vi "LABVIEW做的蓝牙数据发送程序.vi"() -> ()   [LabVIEW 2018]
panel:
  in  "蓝牙设备列表":i32(listbox)
  in  "停止":bool
  out "数据输出":string="SND: AT SP 6\nRCV: AT SP 6\nOK\r\r>SND: AT DP\nRCV: AT DP\nISO 15765-4 (CAN 11/500)\r\r>SND: 01 00\nRCV: 01 00\n41 00 BE 1F B8 10 \r\r>SND: AT H1\nRCV: AT H1\nOK\r\r>SND: 01 00\nRCV: 01 00\n7E1 06 41 00 BE 1F B8 10 \r\r>"
  in  "服务列表":i32(listbox)
  in  "send":bool
  in  "数据输入":string
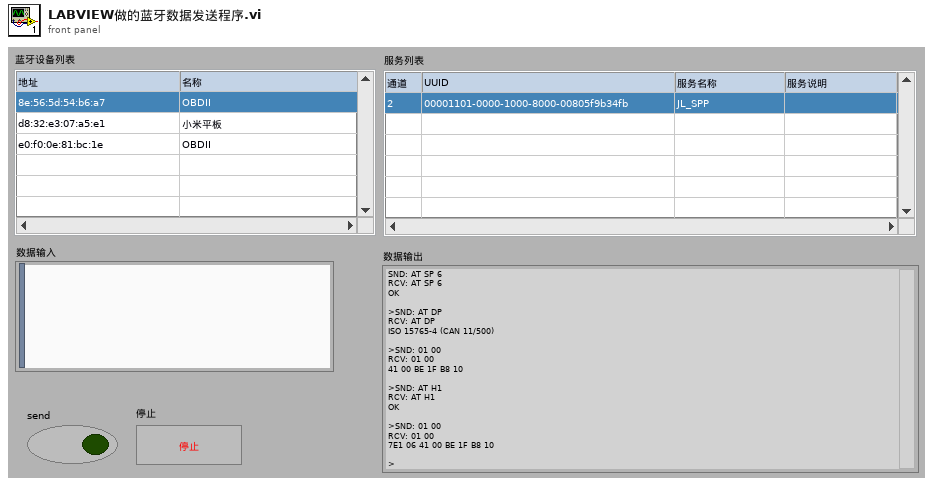
[diagram p1: front panel]
types:
  T1 = cluster{"Address":string, "Device Name":string}[]
  T2 = cluster{"channel":u16, "uuid":string, "service name":string, "service description":string}[]
  T3 = cluster{"channel":u16, "uuid":string, "service name":string, "service description":string}
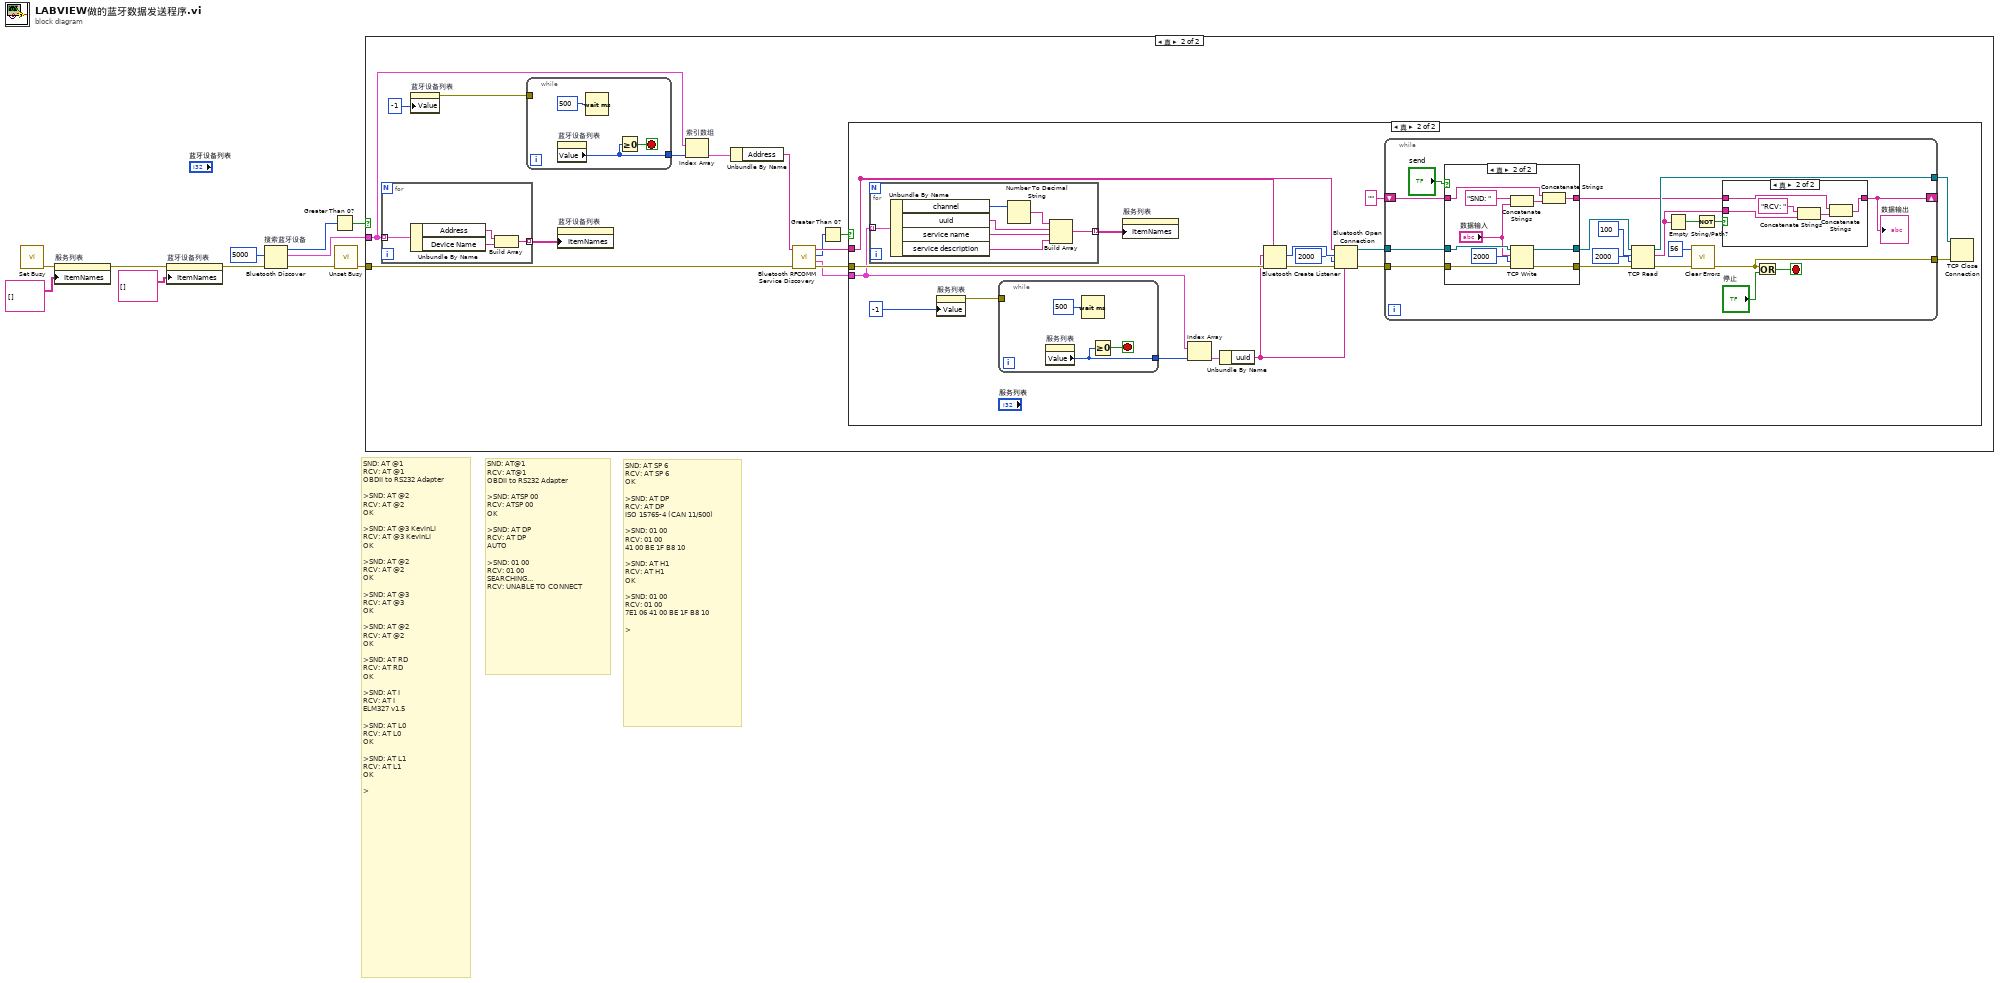
[diagram p0: block diagram]
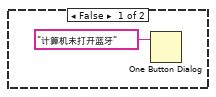
[diagram p2: hidden frame]
diagram:
  # "SND: AT SP 6\nRCV: AT SP 6\nOK\n\n>SND: AT DP\nRCV: AT DP\nISO 15765-4 (CAN 11/500)\n\n>SND: 01 00\nRCV: 01 00\n41 00 BE 1F B8 10 \n\n>SND: AT H1\nRCV: AT H1\nOK\n\n>SND: 01 00\nRCV: 01 00\n7E1 06 41 00 BE 1F B8 10 \n\n>"
  # "SND: AT@1\nRCV: AT@1\nOBDII to RS232 Adapter\n\n>SND: ATSP 00\nRCV: ATSP 00\nOK\n\n>SND: AT DP\nRCV: AT DP\nAUTO\n\n>SND: 01 00\nRCV: 01 00\nSEARCHING...\nRCV: UNABLE TO CONNECT"
  # "SND: AT @1\nRCV: AT @1\nOBDII to RS232 Adapter\n\n>SND: AT @2\nRCV: AT @2\nOK\n\n>SND: AT @3 KevinLi\nRCV: AT @3 KevinLi\nOK\n\n>SND: AT @2\nRCV: AT @2\nOK\n\n>SND: AT @3\nRCV: AT @3\nOK\n\n>SND: AT @2\nRCV: AT @2\nOK\n\n>SND: AT RD\nRCV: AT RD\nOK\n\n>SND: AT I\nRCV: AT I\nELM327 v1.5\n\n>SND: AT L0\nRCV: AT L0\nOK\n\n>SND: AT L1\nRCV: AT L1\nOK\n\n>"
  n1 = call <vilib>:"Set Busy.vi"() -> ("error out"=w3:errorcluster)  [unwired: 10 in, 1 out]
  n2 = property on="服务列表" class="MCListbox (严格)"(error in=w3, "ItemNames"=string[][] [] ("项名")) -> (error out=w4:errorcluster)  [unwired: 1 in, 1 out]
  n3 = property on="蓝牙设备列表" class="MCListbox (严格)"(error in=w4, "ItemNames"=string[][] [] ("项名")) -> (error out=w6:errorcluster)  [unwired: 1 in, 1 out]
  n4 = Bluetooth Discover "搜索蓝牙设备"(8:w6, 10:5000 ("时间限制ms(10000)")) -> (0:w2:errorcluster, 2:w8:T1, 3:w10:u16)
  n5 = Greater Than 0?(x=w10) -> (x > 0?=w9:bool)
  n6 = call <vilib>:"Unset Busy.vi"("error in (no error)"=w2) -> ("error out"=w1:errorcluster)  [unwired: 10 in]
  n7 = case shown="真" w9 {
    tunnel: w1 -> [_ w23]
    tunnel: w8 -> [_ w15]
    frame False {
      n8 = One Button Dialog(message="计算机未打开蓝牙" ("消息")) -> ()  [unwired: 1 in, 1 out]
    }
    frame True {
      n9 = for {
        tunnel: w15 -> [w29] mode=indexing
        tunnel: [w26] -> w17 mode=indexing
        n10 = Unbundle By Name(w29) -> ("Address"=w28:string, "Device Name"=w27:string)
        n11 = Build Array(w28, w27) -> (w26:string[])
      }
      n12 = property on="蓝牙设备列表" class="MCListbox (严格)"("Value"=-1 ("选中行")) -> (error out=w18:errorcluster)  [unwired: 2 in, 1 out]
      n13 = while {
        tunnel: w18 -> [_]
        tunnel: [w30] -> w16
        stop <- w31 stop-if-true
        n14 = property on="蓝牙设备列表" class="MCListbox (严格)"() -> ("Value"=w30:i32)  [unwired: 2 in, 2 out]
        n15 = Wait (ms)(milliseconds to wait=u32 500 ("等待时间（毫秒）")) -> ()  [unwired: 1 out]
        n16 = Greater Or Equal To 0?(x=w30) -> (x >= 0?=w31:bool)
      }
      n17 = property on="蓝牙设备列表" class="MCListbox (严格)"("ItemNames"=w17) -> ()  [unwired: 2 in, 2 out]
      n18 = Index Array "索引数组"(array=w15, index=w16) -> (element=w14:cluster{"Address":string, "Device Name":string})
      n19 = Unbundle By Name(w14) -> ("Address"=w13:string)
      n20 = call <vilib>:"Bluetooth RFCOMM Service Discovery.vi"("error in (no error)"=w23, "address in"=w13) -> ("error out"=w24:errorcluster, "service list"=w20:T2, "number of services"=w22:u16, "address out"=w25:string)  [unwired: 2 in]
      n21 = Greater Than 0?(x=w22) -> (x > 0?=w21:bool)
      n22 = case shown="真" w21 {
        tunnel: w25 -> [_ w46]
        tunnel: w24 -> [_ w45]
        tunnel: w20 -> [_ w36]
        frame False {
        }
        frame True {
          n23 = for {
            tunnel: w36 -> [w56] mode=indexing
            tunnel: [w50] -> w37 mode=indexing
            n24 = Unbundle By Name(w56) -> ("channel"=w55:u16, "uuid"=w53:string, "service name"=w52:string, "service description"=w51:string)
            n25 = Number To Decimal String(number=w55) -> (decimal integer string=w54:string)  [unwired: 1 in]
            n26 = Build Array(w54, w53, w52, w51) -> (w50:string[])
          }
          n27 = property on="服务列表" class="MCListbox (严格)"("Value"=-1 ("选中行")) -> (error out=w34:errorcluster)  [unwired: 2 in, 1 out]
          n28 = while {
            tunnel: w34 -> [_]
            tunnel: [w57] -> w40
            stop <- w58 stop-if-true
            n29 = property on="服务列表" class="MCListbox (严格)"() -> ("Value"=w57:i32)  [unwired: 2 in, 2 out]
            n30 = Wait (ms)(milliseconds to wait=u32 500 ("等待时间（毫秒）")) -> ()  [unwired: 1 out]
            n31 = Greater Or Equal To 0?(x=w57) -> (x >= 0?=w58:bool)
          }
          n32 = property on="服务列表" class="MCListbox (严格)"("ItemNames"=w37) -> ()  [unwired: 2 in, 2 out]
          n33 = Index Array(array=w36, index=w40) -> (element=w38:T3)
          n34 = Unbundle By Name(w38) -> ("uuid"=w39:string)
          n35 = Bluetooth Create Listener(7:w46, 8:w45, 10:w39) -> (0:w49:errorcluster, 2:w48:u16)  [unwired: 1 in, 1 out]
          n36 = Bluetooth Open Connection(6:w39, 8:w49, 9:2000 ("超时毫秒(60000)"), 10:w48, 11:w46) -> (0:w44:errorcluster, 3:w43:refnum<k31>)
          n37 = while {
            tunnel: w44 -> [w78]
            tunnel: w43 -> [w77]
            tunnel: [w74] -> w41
            tunnel: [w68] -> w42
            shift-right: [w60] -> _
            shift-left: "" -> [w65]
            stop <- w66 stop-if-true
            n38 = case shown="真" "send" {
              tunnel: w78 -> [w86 w97]
              tunnel: w77 -> [w87 w96]
              tunnel: [w87 w94] -> w76
              tunnel: [w86 w93] -> w75
              tunnel: w65 -> [w85 w92]
              tunnel: [w85 w88] -> w61
              frame False {
              }
              frame True {
                n39 = Concatenate Strings("SND: " ("字符串"), "数据输入") -> (w91:string)
                n40 = TCP Write(connection ID=w96, data in="数据输入", error in (no error)=w97, 9:2000 ("超时毫秒(25000)")) -> (connection ID out=w94:refnum<k31>, error out=w93:errorcluster)  [unwired: 1 out]
                n41 = Concatenate Strings(w92, w91) -> (w88:string)
              }
            }
            n42 = TCP Read(connection ID=w76, bytes to read=100 ("读取的字节"), error in (no error)=w75, 9:2000 ("超时毫秒(25000)")) -> (connection ID out=w74:refnum<k31>, data out=w62:string, error out=w70:errorcluster)  [unwired: 1 in]
            n43 = Empty String/Path?(string/path=w62) -> (empty?=w64:bool)
            n44 = call <vilib>:"Clear Errors.vi"("error in (no error)"=w70, "specific error code to clear (0: all)"=56) -> ("error out"=w68:errorcluster)  [unwired: 4 in, 1 out]
            n45 = Not(x=w64) -> (.not. x?=w63:bool)
            n46 = case shown="真" w63 {
              tunnel: w62 -> [_ w84]
              tunnel: w61 -> [w79 w82]
              tunnel: [w79 w80] -> w60
              frame False {
              }
              frame True {
                n47 = Concatenate Strings("RCV: " ("字符串"), w84) -> (w81:string)
                n48 = Concatenate Strings(w82, w81) -> (w80:string)
              }
            }
            "数据输出" <- w60
            n49 = Or(x=w68, y="停止") -> (x .or. y?=w66:bool)
          }
          n50 = TCP Close Connection(connection ID=w41, error in (no error)=w42) -> ()  [unwired: 1 in, 2 out]
        }
      }
    }
  }
